vi "Sensor Setting.vi"(8 "error in":errorcluster) -> (0 "error  out":errorcluster)   [LabVIEW 2015]
uses:
  Control Button/Save.ctl
  Control Button/Exit.ctl
  <vilib>/addons/database/Connection.llb/DB Tools Open Connec (String).vi
  Galobal variable_TI.vi
  <vilib>/addons/database/_DB Variant To Data/Database Variant To Data.xnode
  <vilib>/addons/database/NI_Database_API.lvlib
panel:
  out "Lvdt Value(mm)":dbl format="%0.03f"
  out "error out":errorcluster
  in  "String":string
  in  "Cluster 3":T1
  out "Load (N)":dbl format="%0.03f"
  in  "Setting Data":T2 {"LVDT Offset(mm)" format="%0.03f"; "Load Offset" format="%0.03f"; "MaxDistance(mm)" format="%0.02f"; "Min Distance(mm)" format="%0.02f"; "MaxLoad(N)" format="%0.02f"; "Min Load(N)" format="%0.02f"}
  out "Model":string
  in  "Model":string(combo)
  in  "Exit":T3
  in  "Save":T4
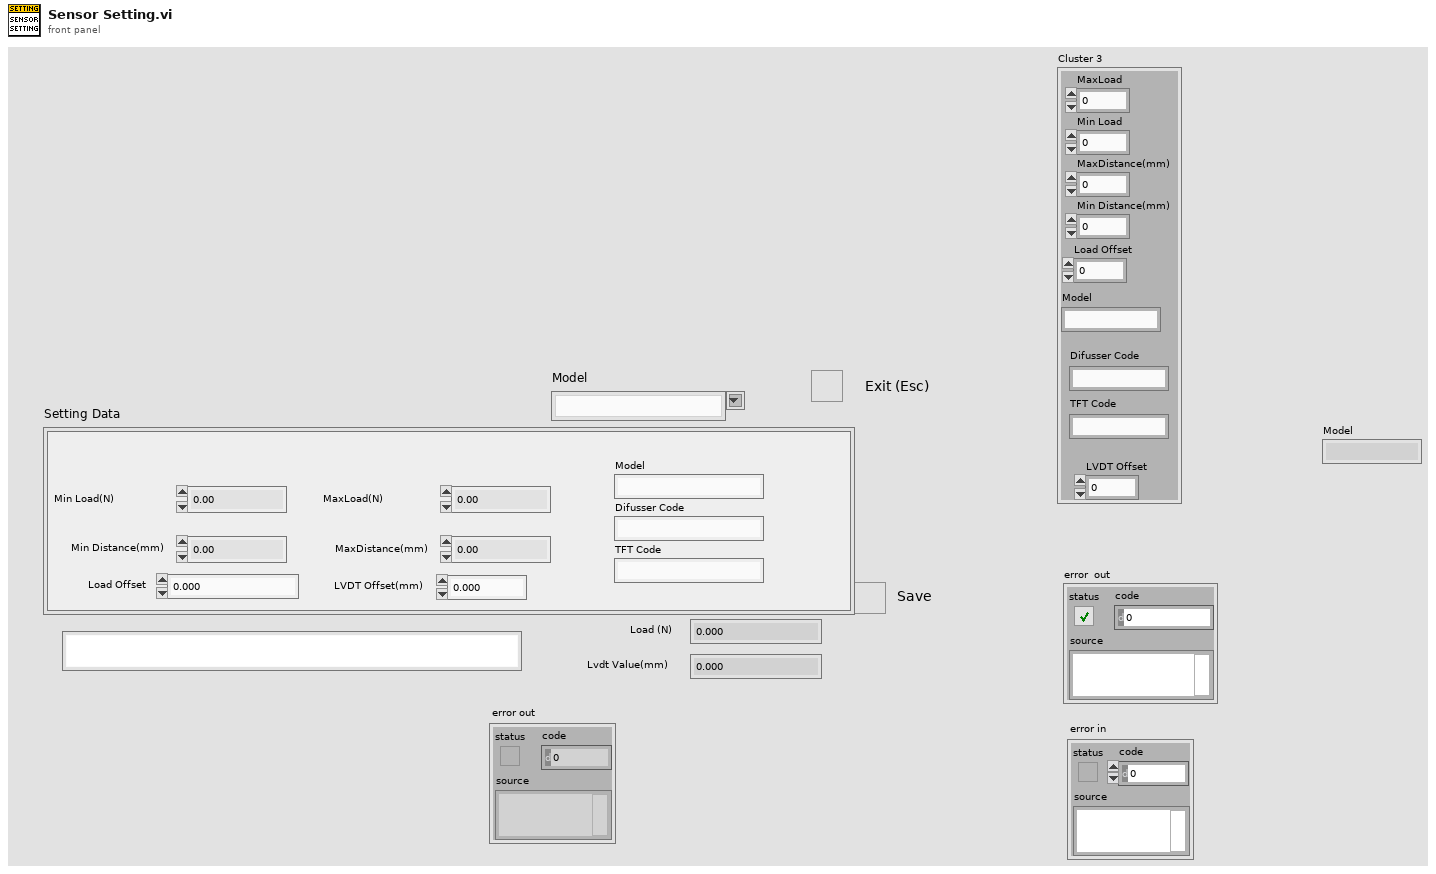
[diagram p1: front panel]
types:
  T1 = cluster{"MaxLoad ":dbl, "Min Load":dbl, "MaxDistance(mm)":dbl, "Min Distance(mm)":dbl, "Load Offset":dbl, "Model":string, "Difusser Code":string, "TFT Code ":string, "LVDT Offset":dbl}
  T2 = cluster{"MaxLoad(N) ":dbl, "Min Load(N)":dbl, "MaxDistance(mm)":dbl, "Min Distance(mm)":dbl, "Load Offset":dbl, "Model":string, "Difusser Code":string, "TFT Code ":string, "LVDT Offset(mm)":dbl}
  T3 = typedef "Exit.ctl" = bool
  T4 = typedef "Save.ctl" = bool
  T5 = typedef "NI_Database_API.lvlib/Conn ObjectReference.ctl" = refnum<k1>
  T6 = cluster{"MaxLoad ":dbl, "Min Load":dbl, "MaxDistance(mm)":dbl, "Min Distance(mm)":dbl, "Load Offset":dbl, "Model":string, "Difusser Code":string, "TFT Code ":string, "Min Distance(mm) 2":dbl}
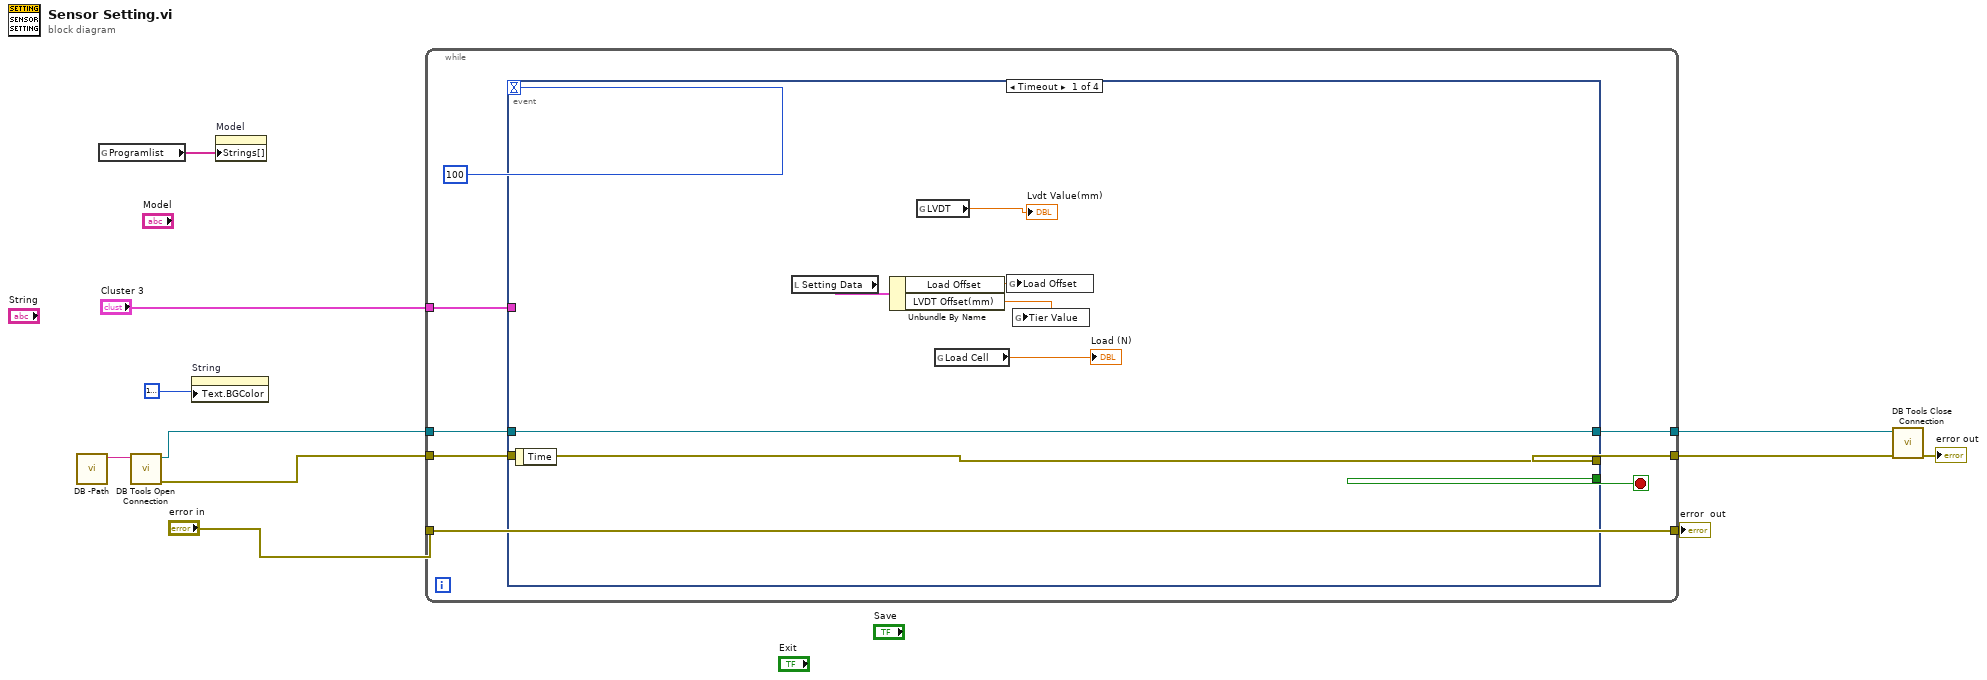
[diagram p0: block diagram]
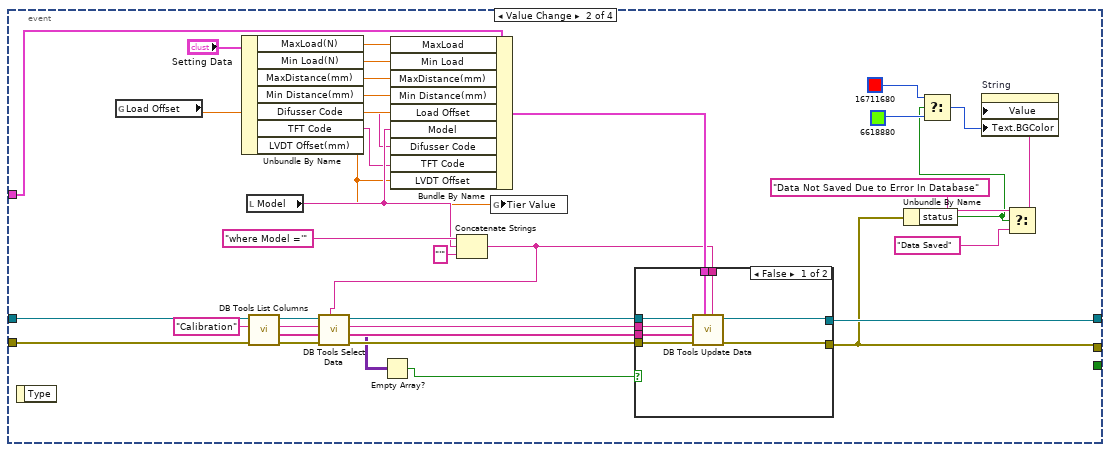
[diagram p2: hidden frame]
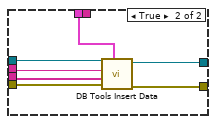
[diagram p3: hidden frame]
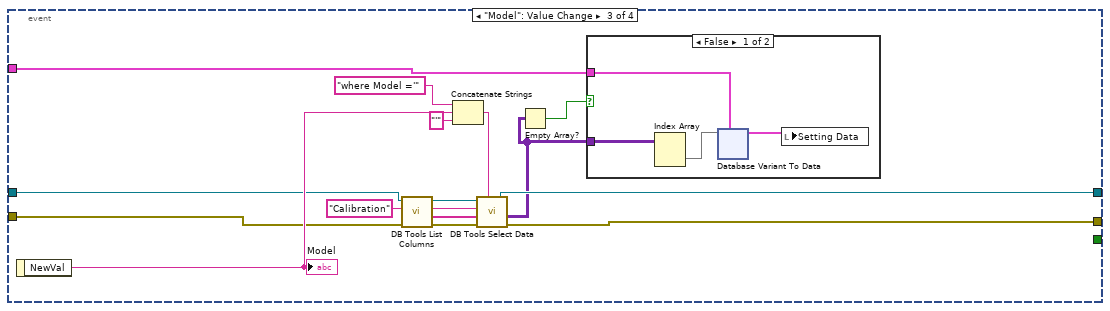
[diagram p4: hidden frame]
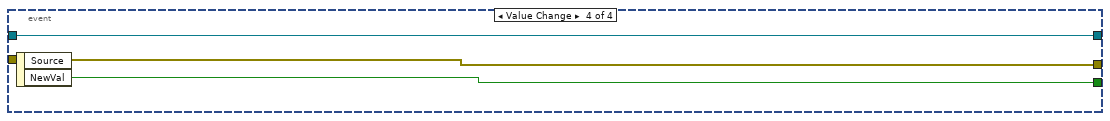
[diagram p6: hidden frame]
diagram:
  n1 = call "DB -Path.vi"() -> ("String"=w11:string)  [unwired: 11 in]
  n2 = global read "Galobal variable_TI.vi" "Programlist"() -> (w6:string[])
  n3 = call-poly <vilib>:"DB Tools Open Connection.vi"("connection information"=w11) -> ("error out"=w9:errorcluster, "connection reference"=w10:T5)  [unwired: 7 in]
  n4 = property on="String" class="Str"("Text.BGColor"=u32 16777226 ("Color Box")) -> ()  [unwired: 2 in, 2 out]
  n5 = property on="Model" class="CmbBox"("Strings[]"=w6) -> ()  [unwired: 2 in, 2 out]
  n6 = while {
    tunnel: w10 -> [w18]
    tunnel: w9 -> [w17]
    tunnel: [w16] -> w8
    tunnel: [w15] -> w7
    tunnel: "error in" -> [w13]
    tunnel: [w13] -> w4
    tunnel: "Cluster 3" -> [w12]
    stop <- w14 stop-if-true
    n7 = event shown="[0] Timeout" {
      selector: _ -> [_ _ _ _]
      dyn-events: _ -> [_ _ _ _]
      timeout: 100 -> [_ _ _ _]
      tunnel: w18 -> [w26 w60 w82 w379]
      tunnel: w17 -> [w25 w59 w81 w380]
      tunnel: [w26 w37 w80 w379] -> w16
      tunnel: [w25 w30 w79 w380] -> w15
      tunnel: [_ _ _ w378] -> w14
      tunnel: w12 -> [_ w48 w78 _]
      event Timeout {
        n8 = event-data() -> ()  [unwired: 1 in, 1 out]
        n9 = local read "Setting Data"() -> (w23:T2)
        n10 = Unbundle By Name(w23) -> ("Load Offset"=w22:dbl, "LVDT Offset(mm)"=w21:dbl)
        n11 = global read "Galobal variable_TI.vi" "LVDT"() -> (→"Lvdt Value(mm)":dbl)
        n12 = global read "Galobal variable_TI.vi" "Load Cell"() -> (→"Load (N)":dbl)
        n13 = global write "Galobal variable_TI.vi" "Load Offset"(w22) -> ()
        n14 = global write "Galobal variable_TI.vi" "Tier Value"(w21) -> ()
      }
      event Value Change {
        w44 = "Calibration" ("table")
        n15 = event-data() -> ()  [unwired: 1 in, 1 out]
        n16 = global read "Galobal variable_TI.vi" "Load Offset"() -> (w49:dbl)
        n17 = Unbundle By Name("Setting Data") -> ("MaxLoad(N)"=w57:dbl, "Min Load(N)"=w56:dbl, "MaxDistance(mm)"=w55:dbl, "Min Distance(mm)"=w54:dbl, "Difusser Code"=w47:string, "TFT Code"=w46:string, "LVDT Offset(mm)"=w27:dbl)
        n18 = local read "Model"() -> (w50:string)
        n19 = call <vilib>:"DB Tools List Columns.vi"("error in (no error)"=w59, "table"=w44, "connection reference"=w60) -> ("error out"=w41:errorcluster, "columns"=w43:string[], "connection reference out"=w45:T5)  [unwired: 1 in, 1 out]
        n20 = Bundle By Name(cluster=w48, "MaxLoad"=w57, "Min Load"=w56, "MaxDistance(mm)"=w55, "Min Distance(mm)"=w54, "Load Offset"=w49, "Model"=w50, "Difusser Code"=w47, "TFT Code"=w46, "LVDT Offset"=w27) -> (w53:T1)
        n21 = Concatenate Strings("where Model ='" ("string"), w50, "'" ("string")) -> (w28:string)
        n22 = call <vilib>:"DB Tools Select Data.vi"("condition"=w28, "error in (no error)"=w41, "columns"=w43, "table"=w44, "connection reference"=w45) -> ("error out"=w40:errorcluster, "data"=w39:variant[][], "connection reference out"=w42:T5)  [unwired: 1 in]
        n23 = Empty Array?(array=w39) -> (empty?=w38:bool)
        n24 = global write "Galobal variable_TI.vi" "Tier Value"(w27) -> ()
        n25 = case shown="False" w38 {
          tunnel: w40 -> [w68 w74]
          tunnel: w42 -> [w67 w75]
          tunnel: w43 -> [w66 w72]
          tunnel: w53 -> [w65 w71]
          tunnel: w28 -> [w64 _]
          tunnel: w44 -> [w63 w73]
          tunnel: [w62 w70] -> w37
          tunnel: [w61 w69] -> w30
          frame False {
            n26 = call <vilib>:"DB Tools Update Data.vi"("condition"=w64, "data"=w65, "error in (no error)"=w68, "columns"=w66, "table"=w63, "connection reference"=w67) -> ("error out"=w61:errorcluster, "connection reference out"=w62:T5)  [unwired: 4 in]
          }
          frame True {
            n27 = call <vilib>:"DB Tools Insert Data.vi"("data"=w71, "error in (no error)"=w74, "columns"=w72, "table"=w73, "connection reference"=w75) -> ("error out"=w69:errorcluster, "connection reference out"=w70:T5)  [unwired: 5 in]
          }
        }
        n28 = Unbundle By Name(w30) -> ("status"=w29:bool)
        n29 = Select(t=u32 16711680 ("Color Box"), s=w29, f=u32 6618880 ("Color Box")) -> (s? t:f=w31:u32)
        n30 = Select(t="Data Not Saved Due to Error In Database", s=w29, f="Data Saved") -> (s? t:f=w34:string)
        n31 = property on="String" class="Str"("Value"=w34, "Text.BGColor"=w31) -> ()  [unwired: 2 in, 2 out]
      }
      event "Model": Value Change {
        w84 = "Calibration" ("table")
        n32 = event-data() -> ("NewVal"=w83:string)  [unwired: 1 in]
        "Model" <- w83
        n33 = call <vilib>:"DB Tools List Columns.vi"("error in (no error)"=w81, "table"=w84, "connection reference"=w82) -> ("error out"=w90:errorcluster, "columns"=w88:string[], "connection reference out"=w89:T5)  [unwired: 1 in, 1 out]
        n34 = Concatenate Strings("where Model ='" ("string"), w83, "'" ("string")) -> (w85:string)
        n35 = call <vilib>:"DB Tools Select Data.vi"("condition"=w85, "error in (no error)"=w90, "columns"=w88, "table"=w84, "connection reference"=w89) -> ("error out"=w79:errorcluster, "data"=w77:variant[][], "connection reference out"=w80:T5)  [unwired: 1 in]
        n36 = Empty Array?(array=w77) -> (empty?=w76:bool)
        n37 = case shown="False" w76 {
          tunnel: w77 -> [w94 _]
          tunnel: w78 -> [w92 _]
          frame False {
            n38 = Index Array(array=w94) -> (element=w93:variant[])  [unwired: 2 in]
            n39 = xnode "Database Variant To Data"("database variant"=w93, "type"=w92) -> ("data"=w91:T6)  [unwired: 1 in, 1 out]
            n40 = local write "Setting Data"(w91) -> ()
          }
          frame True {
          }
        }
      }
      event Value Change {
        n41 = event-data() -> ("NewVal"=w378:T3)  [unwired: 1 in, 1 out]
      }
    }
  }
  "error  out" <- w4
  n42 = call <vilib>:"DB Tools Close Connection.vi"("error in (no error)"=w7, "connection reference"=w8) -> ("error out"=→"error out":errorcluster)  [unwired: 5 in]
